vi "iWorx - Thermistor.vi"() -> ()   [LabVIEW 2012]
uses:
  <vilib>/DAQmx/read.llb/DAQmx Read (Analog 1D DBL NChan 1Samp).vi
  <vilib>/DAQmx/create/channels.llb/DAQmx Create Channel (AI-Voltage-Basic).vi
  <vilib>/DAQmx/miscellaneous.llb/DAQmx Fill In Error Info.vi
panel:
  in  "Set Up":bool
  in  "Set Value":dbl min=-100.0 max=300.0 step=0.1 format="%#_g°C"
  in  "Set":bool
  in  "Calibration Coefficients":cluster{"Ka":dbl, "Kb":dbl, "Kc":dbl}={"Ka"=0.00073998, "Kb"=0.00027874, "Kc"=9.2632e-08}
  in  "Channel":u16(ring) items=["Channel 1", "Channel 2"]
  in  "Pause Button":bool
  in  "Snapshot":bool
  out "Processed Signal":dbl(knob) caption="Temperature" scale=0.0..100.0
  in  "stop":bool
  out "Waveform Chart":dbl(graph)
  in  "Sample Timing":u16(ring)=200 items=["20Hz"=50, "5 Hz"=200, "2 Hz"=500, "1 Hz"=1000, ".5 Hz"=2000, ".2 Hz"=5000]
  in  "Clear Chart":bool
  in  "Open Log":bool
  in  "Autoscale Y":bool=TRUE
  out "Raw Signal":dbl(knob) scale=-4.0..1.0
  # "iWorx - Thermistor - Data Logger"
  # "Sensor Input"
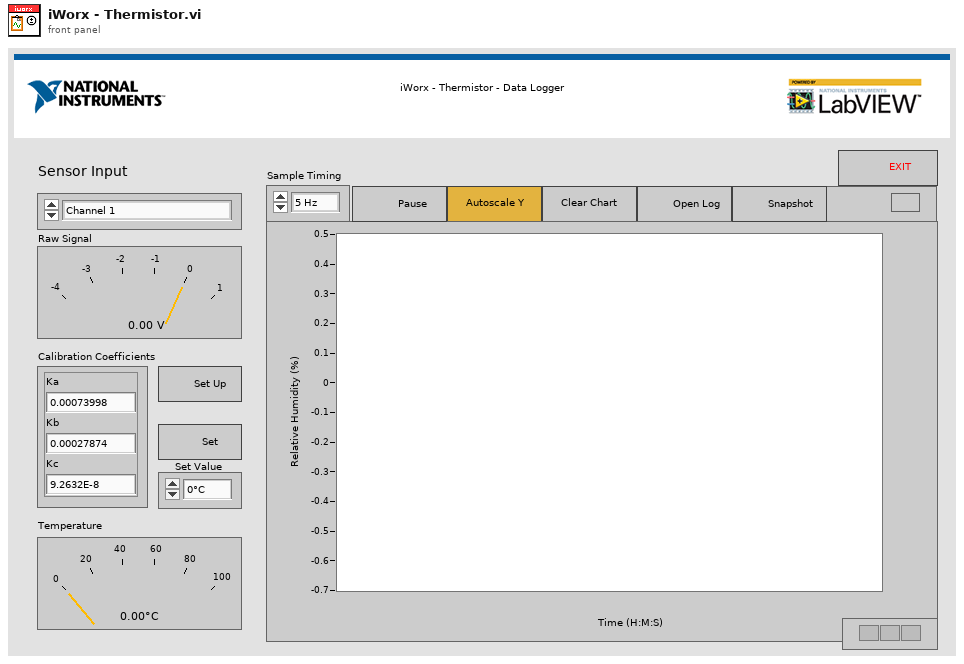
[diagram p1: front panel]
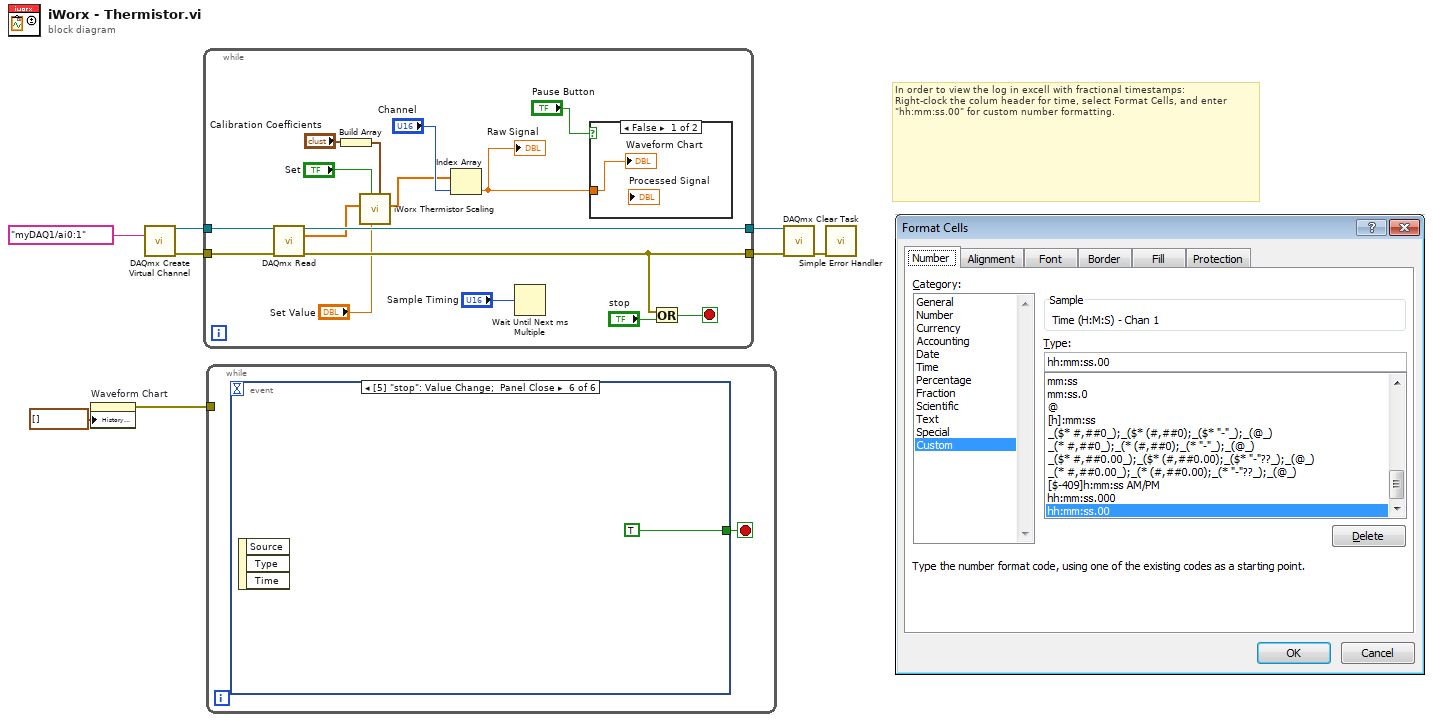
[diagram p0: block diagram]
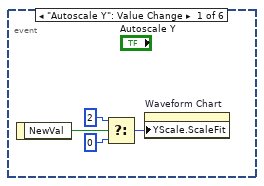
[diagram p2: hidden frame]
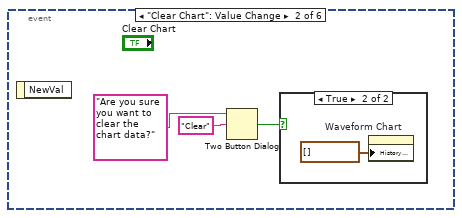
[diagram p3: hidden frame]
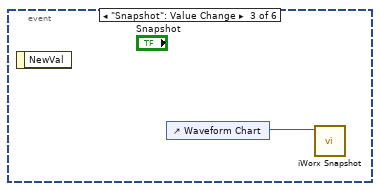
[diagram p5: hidden frame]
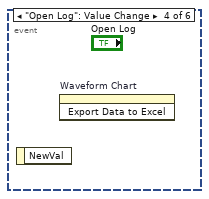
[diagram p6: hidden frame]
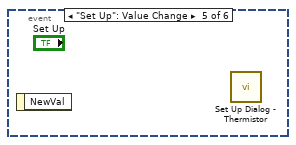
[diagram p7: hidden frame]
diagram:
  # "In order to view the log in excell with fractional timestamps: \nRight-clock the colum header for time, select Format Cells, and enter \"hh:mm:ss.00\" for custom number formatting."
  n1 = property on="Waveform Chart" class="WFChart (strict)"("History Data"=waveform(dbl)[] []) -> (error out=w3:errorcluster)  [unwired: 2 in, 1 out]
  n2 = call-poly <vilib>:"DAQmx Create Virtual Channel.vi"("physical channels"=tag "myDAQ1/ai0:1") -> ("task out"=w5:refnum<k21>, "error out"=w4:errorcluster)  [unwired: 13 in]
  n3 = while {
    tunnel: w5 -> [w22]
    tunnel: [w21] -> w8
    tunnel: w4 -> [w20]
    tunnel: [w18] -> w7
    stop <- w19 stop-if-true
    n4 = call-poly <vilib>:"DAQmx Read.vi"("task/channels in"=w22, "error in"=w20) -> ("task out"=w21:refnum<k21>, "data"=w15:dbl[], "error out"=w18:errorcluster)  [unwired: 11 in]
    n5 = Build Array("Calibration Coefficients") -> (w14:cluster{"Ka":dbl, "Kb":dbl, "Kc":dbl}[])
    n6 = call "iWorx Thermistor Scaling.vi"("Calibration Coefficients"=w14, "Set Point Temp"="Set Value", "Set"="Set", "Vt Measured"=w15) -> ("Temps"=w12:dbl[])  [unwired: 6 in, 1 out]
    n7 = Index Array(array=w12, index="Channel") -> (element=w11:dbl)
    "Raw Signal" <- w11
    n8 = Wait Until Next ms Multiple(millisecond multiple="Sample Timing") -> ()  [unwired: 1 out]
    n9 = case shown="False" "Pause Button" {
      tunnel: w11 -> [w25 _]
      frame False {
        "Waveform Chart" <- w25
      }
      frame True {
      }
    }
    n10 = Or(x=w18, y="stop") -> (x .or. y?=w19:bool)
  }
  n11 = while {
    tunnel: w3 -> [_]
    stop <- w26 stop-if-true
    n12 = event shown="[5] \"stop\": Value Change;  Panel Close" {
      selector: _ -> [_ _ _ _ _ _]
      dyn-events: _ -> [_ _ _ _ _ _]
      timeout: _ -> [_ _ _ _ _ _]
      tunnel: [_ _ _ _ _ TRUE] -> w26
      event "Autoscale Y": Value Change {
        n13 = event-data() -> ("NewVal"=w28:bool)  [unwired: 1 in]
        n14 = Select(t=u8 2 ("Y Scale.Scale Fit"), s=w28, f=u8 0 ("Y Scale.Scale Fit")) -> (s? t:f=w27:u8)
        n15 = property on="Waveform Chart" class="WFChart (strict)"("YScale.ScaleFit"=w27) -> ()  [unwired: 2 in, 2 out]
      }
      event "Clear Chart": Value Change {
        n16 = event-data() -> ()  [unwired: 1 in, 1 out]
        n17 = Two Button Dialog(message="Are you sure you want to clear the chart data?", 2:"Clear" ("T button name (\"OK\")")) -> (T button?=w32:bool)  [unwired: 1 in]
        n18 = case shown="True" w32 {
          frame False {
          }
          frame True {
            n19 = property on="Waveform Chart" class="WFChart (strict)"("History Data"=waveform(dbl)[] []) -> ()  [unwired: 2 in, 2 out]
          }
        }
      }
      event "Snapshot": Value Change {
        n20 = event-data() -> ()  [unwired: 1 in, 1 out]
        n21 = control-ref of="Waveform Chart"() -> (w35:refnum<vi>)
        n22 = call "iWorx Snapshot.vi"("WaveformChart in"=w35) -> ()  [unwired: 10 in, 1 out]
      }
      event "Open Log": Value Change {
        n23 = event-data() -> ()  [unwired: 1 in, 1 out]
        n24 = invoke on="Waveform Chart" class="WFChart (strict)" method="Export Data to Excel"() -> ()  [unwired: 3 in, 3 out]
      }
      event "Set Up": Value Change {
        n25 = event-data() -> ()  [unwired: 1 in, 1 out]
        n26 = call "Set Up Dialog - Thermistor.vi"() -> ()  [unwired: 12 in]
      }
      event "stop": Value Change; Panel Close {
        n27 = event-data() -> ()  [unwired: 1 in, 3 out]
      }
    }
  }
  n28 = call <vilib>:"DAQmx Clear Task.vi"("task in"=w8, "error in"=w7) -> ("error out"=w2:errorcluster)  [unwired: 13 in]
  n29 = call <vilib>:"Simple Error Handler.vi"("error in (no error)"=w2) -> ()  [unwired: 4 in, 5 out]
